vi "Flatten JSON Object to JSONpath Array.vi"(6 "Initial Path":string="$", 11 "JSON":string) -> (1 "<JSON>":string[](array[string]) caption="<JSON>Items", 3 "$Paths":string[](array[string]))   [LabVIEW 2017, in "JSONtext.lvlib"]
doc: "Takes a JSON Value and \"flattens\" the Object structure, producing out arrays of the $Paths to each item and the corresponding items. This works recursively on all subObjects.\n\nFor example: the JSON {\"A\":{\"B1\":1\"B2:\"x\"},\"A2\":true,\"A3\":{\"C\":123}} produces the arrays:\n$Paths (Items):\n$.A.B1 (1)\n$.A.B2 (\"x\")\n$.A2 (true)\n$.A3.C (123)"
uses:
  JSONtext.lvlib
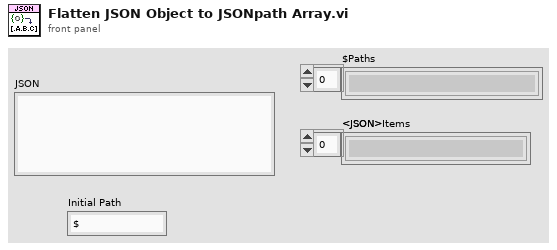
[diagram p1: front panel]
types:
  T1 = typedef "JSONtext.lvlib/JSON Value Type.ctl" = enum16{"Not a JSON Value", "JSON Object", "JSON Array", "String", "Number", "true", "false", "null"}
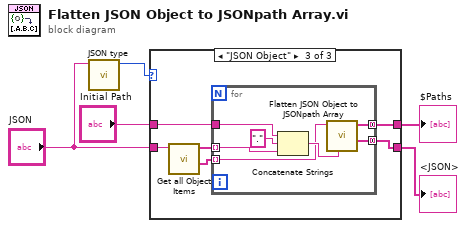
[diagram p0: block diagram]
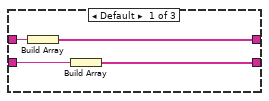
[diagram p2: hidden frame]
diagram:
  n1 = call "JSON type.vi"("JSON"="JSON") -> ("JSON Value Type"=w1:T1)  [unwired: 9 in, 1 out]
  n2 = case shown="\"JSON Object\"" w1 {
    tunnel: "JSON" -> [w9 _ w15]
    tunnel: [w6 _ w13] -> w2
    tunnel: [w8 _ w10] -> w3
    tunnel: "Initial Path" -> [w7 _ w14]
    frame Default {
      n3 = Build Array(w7) -> (w6:string[])
      n4 = Build Array(w9) -> (w8:string[])
    }
    frame "Not a JSON Value" {
    }
    frame "JSON Object" {
      n5 = call "Get all Object Items.vi"("JSON"=w15) -> ("<JSON>"=w11:string[], "Item Names"=w12:string[])  [unwired: 7 in, 2 out]
      n6 = for {
        tunnel: w14 -> [w22]
        tunnel: [w19] -> w13 mode=concatenating
        tunnel: w12 -> [w20] mode=indexing
        tunnel: w11 -> [w17] mode=indexing
        tunnel: [w16] -> w10 mode=concatenating
        n7 = Concatenate Strings(w22, "." ("string"), w20) -> (w18:string)
        n8 = call "Flatten JSON Object to JSONpath Array.vi"("Initial Path"=w18, "JSON"=w17) -> ("<JSON>"=w16:string[], "$Paths"=w19:string[])  [unwired: 8 in]
      }
    }
  }
  "<JSON>" <- w3
  "$Paths" <- w2
